vi "Auto_Routine_DepositHighBackup.vi"(8 "error in (no error)":errorcluster) -> (0 "error out":errorcluster)   [LabVIEW 2023]
doc: "Deposits a cone on the upper node then backs up\nInputs: \n--ErrorIn--\nOutputs:\n--ErrorOut--"
uses:
  Arm/ArmGamePiecePreset.ctl
  Arm/ArmPositionPreset.ctl
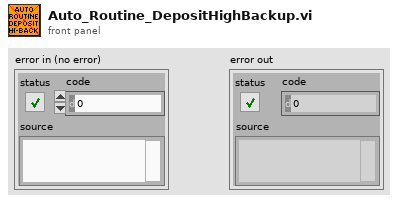
[diagram p1: front panel]
types:
  T1 = typedef "ArmGamePiecePreset.ctl" = enum16{"Cube", "Cone"}
  T2 = typedef "ArmPositionPreset.ctl" = enum16{"Upper", "Lower", "Middle", "Home", "Shelf", "Floor", "HalfFloor", "HalfHome"}
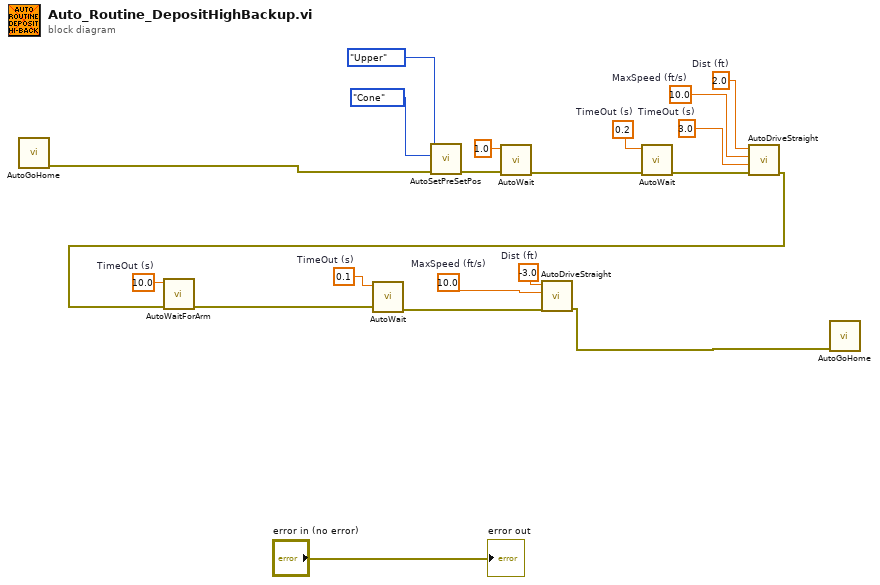
[diagram p0: block diagram]
diagram:
  w18 = 10.0  # MaxSpeed (ft/s)
  w17 = 3.0  # TimeOut (s)
  w16 = 10.0  # MaxSpeed (ft/s)
  w15 = 2.0  # Dist (ft)
  w13 = -3.0  # Dist (ft)
  w12 = 0.1  # TimeOut (s)
  w11 = 0.2  # TimeOut (s)
  w10 = 10.0  # TimeOut (s)
  n1 = call "AutoGoHome.vi"() -> ("error out"=w2:errorcluster)  [unwired: 11 in]
  n2 = call "AutoSetPreSetPos.vi"("error in (no error)"=w2, "Game Piece"=ArmGamePiecePreset."Cone", "Position"=ArmPositionPreset."Upper") -> ("error out"=w19:errorcluster)  [unwired: 8 in]
  n3 = call "AutoWait.vi"("error in (no error)"=w19, "TimeOut (s)"=1.0) -> ("error out"=w3:errorcluster)  [unwired: 9 in]
  n4 = call "AutoWait.vi"("error in (no error)"=w3, "TimeOut (s)"=w11) -> ("error out"=w8:errorcluster)  [unwired: 9 in]
  n5 = call "AutoDriveStraight.vi"("error in (no error)"=w8, "TimeOut (s)"=w17, "MaxSpeed (ft/s)"=w16, "Dist (ft)"=w15) -> ("error out"=w9:errorcluster)  [unwired: 7 in]
  n6 = call "AutoWaitForArm.vi"("error in (no error)"=w9, "TimeOut (s)"=w10) -> ("error out"=w1:errorcluster)  [unwired: 9 in]
  n7 = call "AutoWait.vi"("error in (no error)"=w1, "TimeOut (s)"=w12) -> ("error out"=w14:errorcluster)  [unwired: 9 in]
  n8 = call "AutoDriveStraight.vi"("error in (no error)"=w14, "MaxSpeed (ft/s)"=w18, "Dist (ft)"=w13) -> ("error out"=w4:errorcluster)  [unwired: 8 in]
  n9 = call "AutoGoHome.vi"("error in (no error)"=w4) -> ()  [unwired: 10 in, 1 out]
  "error out" <- "error in (no error)"
